vi "Init.vi"(8 "Error In":errorcluster, 11 "reference in":refnum<class "Thermometer Multichannel.lvclass">) -> (0 "Error Out":errorcluster, 3 "reference out":refnum<class "Thermometer Multichannel.lvclass">)   [LabVIEW 2024, in "Thermometer Multichannel.lvclass"]
uses:
  Thermometer Multichannel.lvclass
  Interfaces/IConfigure/IConfigure.lvclass
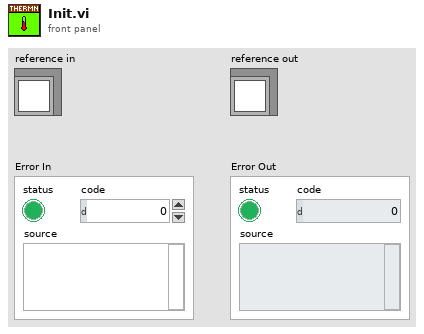
[diagram p1: front panel]
types:
  T1 = typedef "Thermometer Multichannel.lvclass/ObjectAttributes.ctl" = cluster{"IConfigure":refnum<class "IConfigure.lvclass">, "Worker Enqueuer":refnum<class "Message Enqueuer.lvclass">}
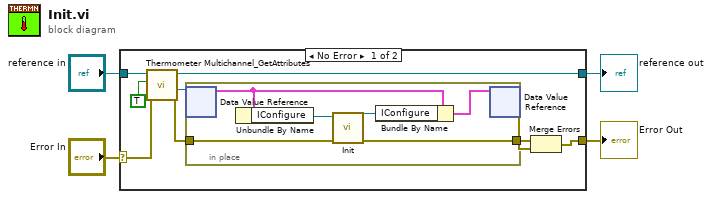
[diagram p0: block diagram]
diagram:
  n1 = case shown="No Error" "Error In" {
    selector: "Error In" -> [w13 w21]
    tunnel: [w6 w21] -> w3
    tunnel: [w11 w20] -> w1
    tunnel: "reference in" -> [w12 w20]
    frame No Error {
      n2 = call "Thermometer Multichannel_GetAttributes.vi"("Error In"=w13, "OnlyGetDvrReference(False)"=TRUE, "reference in"=w12) -> ("Error Out"=w10:errorcluster, "DataRef"=w7:refnum<data-value>, "reference out"=w11:refnum<class "Thermometer Multichannel.lvclass">)  [unwired: 5 in, 1 out]
      n3 = in-place {
        in-place-border: w10 -> [w19]
        in-place-border: [w18] -> w9
        n4 = in-place-dvr #1(w7) -> (w15:T1)  [unwired: 1 out]
        n5 = Unbundle By Name(w15) -> ("IConfigure"=w17:refnum<class "IConfigure.lvclass">)
        n6 = call-dynamic "Init.vi"("error in"=w19, "IInitialize in"=w17) -> ("error out"=w18:errorcluster, "IInitialize out"=w16:refnum<class "IConfigure.lvclass">)  [unwired: 8 in]
        n7 = Bundle By Name(cluster=w15, "IConfigure"=w16) -> (w14:T1)
        n8 = in-place-dvr #1(w14) -> (w5:errorcluster)  [unwired: 1 out]
      }
      n9 = Merge Errors(w9, w5) -> (w6:errorcluster)
    }
    frame Error {
    }
  }
  "Error Out" <- w3
  "reference out" <- w1
